vi "CalcSelection.vi"(10 "Before":string, 11 "Line Number":i32) -> (2 "Exists":bool, 3 "Cluster":cluster{i32, i32})   [LabVIEW 2016]
panel:
  in  "Start Offset":i32
  out "Area of error":string
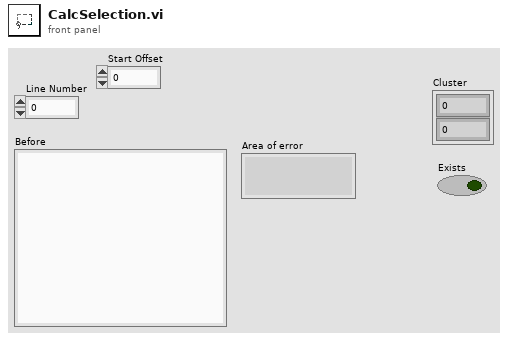
[diagram p1: front panel]
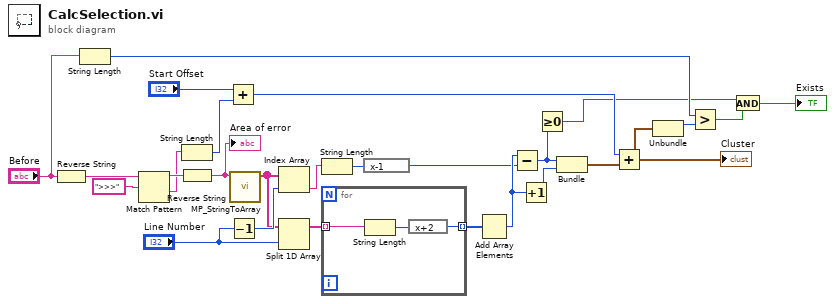
[diagram p0: block diagram]
diagram:
  n1 = Reverse String(1:"Before") -> (0:w16:string)
  n2 = String Length(string="Before") -> (length=w4:i32)
  n3 = Match Pattern(string=w16, regular expression=">>>") -> (before substring=w18:string, after substring=w14:string)  [unwired: 1 in, 2 out]
  n4 = String Length(string=w14) -> (length=w13:i32)
  n5 = Reverse String(1:w18) -> (0:w19:string)
  "Area of error" <- w19
  n6 = Add(x="Start Offset", y=w13) -> (x+y=w11:i32)
  n7 = Decrement(x="Line Number") -> (x-1=w24:i32)
  n8 = call "MP_StringToArray.vi"("write buffer"=w19) -> ("Array"=w23:string[])  [unwired: 10 in]
  n9 = Index Array(array=w23, index=w24) -> (element=w22:string)
  n10 = Split 1D Array(array=w23, index="Line Number") -> (first subarray=w25:string[])  [unwired: 1 out]
  n11 = String Length(string=w22) -> (length=w20:i32)
  n12 = for {
    tunnel: w25 -> [w29] mode=indexing
    tunnel: [w28] -> w26 mode=indexing
    n13 = String Length(string=w29) -> (length=w30:i32)
    n14 = expression code="x+2"(w30) -> (w28:i32)
  }
  n15 = expression code="x-1"(w20) -> (w21:i32)
  n16 = Add Array Elements(numeric array=w26) -> (sum=w27:i32)
  n17 = Subtract(x=w27, y=w21) -> (x-y=w8:i32)
  n18 = Increment(x=w27) -> (x+1=w9:i32)
  n19 = Greater Or Equal To 0?(x=w8) -> (x >= 0?=w2:bool)
  n20 = Bundle(w8, w9) -> (w10:cluster{i32, i32})  [unwired: 1 in]
  n21 = Add(x=w11, y=w10) -> (x+y=w6:cluster{i32, i32})
  "Cluster" <- w6
  n22 = Unbundle(w6) -> (w5:i32)  [unwired: 1 out]
  n23 = Greater?(x=w4, y=w5) -> (0:w3:bool)
  n24 = And(x=w2, y=w3) -> (x .and. y?=→"Exists":bool)
